vi "SpinnerMotorValue.vi"() -> ()   [LabVIEW 2016]
panel:
  out "SpinnerMotorValue":dbl
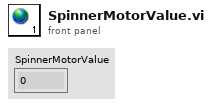
[diagram p1: front panel]
diagram:
